vi "Find Peaks v2.vi"(9 "Exclusivity Width (Hz)":dbl, 10 "Power Spectrum":waveform(dbl), 11 "#Peaks to Locate":i32) -> (3 "Array":dbl[](array[numeric]))   [LabVIEW 2023]
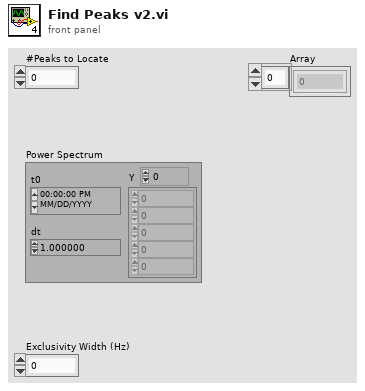
[diagram p1: front panel]
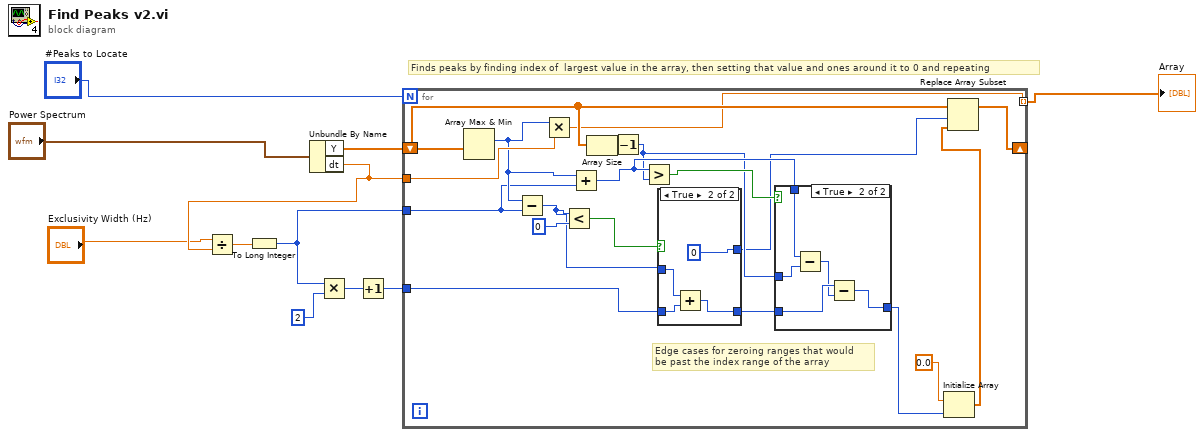
[diagram p0: block diagram]
diagram:
  # "Finds peaks by finding index of  largest value in the array, then setting that value and ones around it to 0 and repeating"
  n1 = Unbundle By Name("Power Spectrum") -> ("Y"=w8:dbl[], "dt"=w2:dbl)
  n2 = Divide(x="Exclusivity Width (Hz)", y=w2) -> (x/y=w3:dbl)
  n3 = To Long Integer(number=w3) -> (32bit integer=w9:i32)
  n4 = Multiply(x=w9, y=2) -> (x*y=w5:i32)
  n5 = Increment(x=w5) -> (x+1=w7:i32)
  n6 = for {
    N: "#Peaks to Locate" -> [_]
    tunnel: w2 -> [w29]
    tunnel: w7 -> [w25]
    tunnel: w9 -> [w21]
    shift-right: [w13] -> _
    shift-left: w8 -> [w22]
    tunnel: [w12] -> w10 mode=indexing
    # "Edge cases for zeroing ranges that would\nbe past the index range of the array"
    n7 = Array Max & Min(array=w22) -> (max index (indices)=w23:i32)  [unwired: 3 out]
    n8 = Subtract(x=w23, y=w21) -> (x-y=w24:i32)
    n9 = Multiply(x=w23, y=w29) -> (x*y=w12:dbl)
    n10 = Less?(x=w24, y=0) -> (x < y?=w26:bool)
    n11 = Add(x=w23, y=w21) -> (x+y=w17:i32)
    n12 = Array Size(array=w22) -> (size(s)=w20:i32)
    n13 = Decrement(x=w20) -> (x-1=w16:i32)
    n14 = Greater?(x=w17, y=w16) -> (0:w19:bool)
    n15 = case shown="True" w26 {
      tunnel: w25 -> [w37 w42]
      tunnel: w24 -> [w38 w41]
      tunnel: [w38 0] -> w14
      tunnel: [w37 w39] -> w18
      frame False {
      }
      frame True {
        n16 = Add(x=w41, y=w42) -> (x+y=w39:i32)
      }
    }
    n17 = case shown="True" w19 {
      tunnel: w18 -> [w31 w36]
      tunnel: [w31 w34] -> w15
      tunnel: w17 -> [_ w33]
      tunnel: w16 -> [_ w32]
      frame False {
      }
      frame True {
        n18 = Subtract(x=w33, y=w32) -> (x-y=w35:i32)
        n19 = Subtract(x=w36, y=w35) -> (x-y=w34:i32)
      }
    }
    n20 = Initialize Array(0.0 ("element"), w15) -> (w28:dbl[])
    n21 = Replace Array Subset(array=w22, new element=w28, index=w14) -> (w13:dbl[])
  }
  "Array" <- w10
